vi "PC_DFM_Single.vi"() -> ()   [LabVIEW 2021]
uses:
  Digital Frequency Measurement/Typedefs/Range Settings.ctl
  Digital Frequency Measurement/DAQ_Digital Frequency Measurement.lvlib
panel:
  out "error out":errorcluster
  out "Detected Frequency (Hz)":dbl=10000.0 format="%.6p"
  in  "Input Frequency Divisor":u32=4 min=4 step=1
  in  "Range Settings":T1={"Max Frequency (Hz)"=20000000.0, "Min Frequency (Hz)"=1.0} {"Min Frequency (Hz)" format="%.6p"; "Max Frequency (Hz)" format="%.6p"}
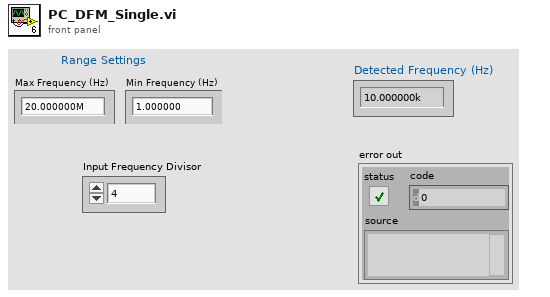
[diagram p1: front panel]
types:
  T1 = typedef "DAQ_Digital Frequency Measurement.lvlib/Range Settings.ctl" = cluster{"Max Frequency (Hz)":dbl, "Min Frequency (Hz)":dbl}
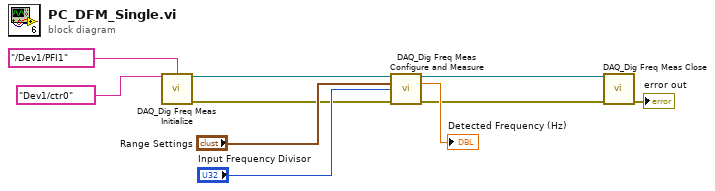
[diagram p0: block diagram]
diagram:
  n1 = call "DAQ_Dig Freq Meas Initialize.vi"("Physical Channel (counter)"=tag "Dev1/ctr0", "Input Terminal"=tag "/Dev1/PFI1") -> ("DAQmx Task Out"=w8:refnum<k21>, "error out"=w2:errorcluster)  [unwired: 12 in]
  n2 = call "DAQ_Dig Freq Meas Configure and Measure.vi"("DAQmx Task In"=w8, "Range Settings"="Range Settings", "Input Frequency Divisor"="Input Frequency Divisor", "error in"=w2) -> ("DAQmx Task Out"=w7:refnum<k21>, "Detected Frequency (Hz)"=→"Detected Frequency (Hz)":dbl, "error out"=w1:errorcluster)  [unwired: 9 in]
  n3 = call "DAQ_Dig Freq Meas Close.vi"("DAQmx Task In"=w7, "error in"=w1) -> ("error out"=→"error out":errorcluster)  [unwired: 13 in]
